vi "Read Temperature.vi"(0 "Session Handle in":T1, 11 "error in (no error)":errorcluster) -> (4 "Session Handle out":T1, 6 "Temperature":dbl, 8 "Success?":bool, 10 "Error Code":string, 15 "error out":errorcluster)   [LabVIEW 2015, in "PAS.lvclass"]
uses:
  PAS.lvclass
  Typedefs/Session Handle.ctl
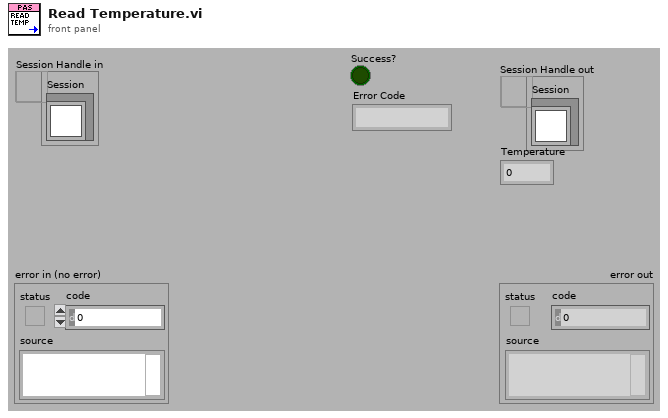
[diagram p1: front panel]
types:
  T1 = typedef "PAS.lvclass/Session Handle.ctl" = refnum<data-value>
  T2 = typedef "XNET Frame CAN.ctl" = cluster{"timestamp":timestamp, "payload":u8[], "identifier":u32, "type":T3, "extended?":bool, "echo?":bool}
  T3 = typedef "XNET Frame Type CAN.ctl" = u8
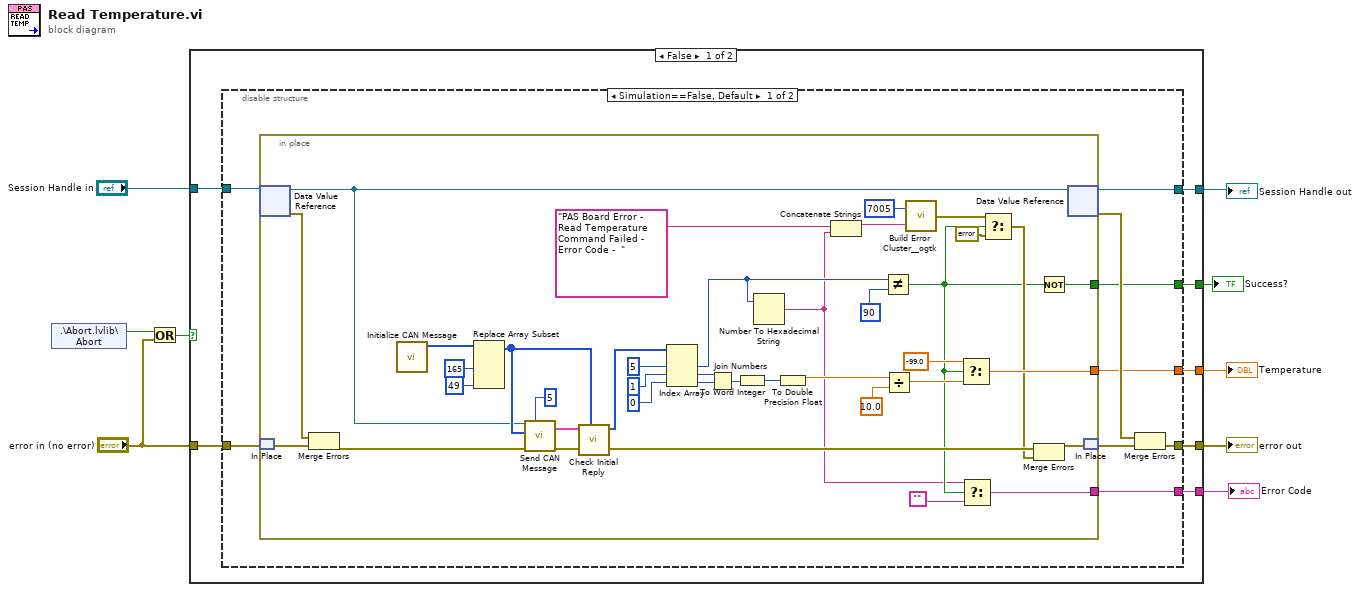
[diagram p0: block diagram]
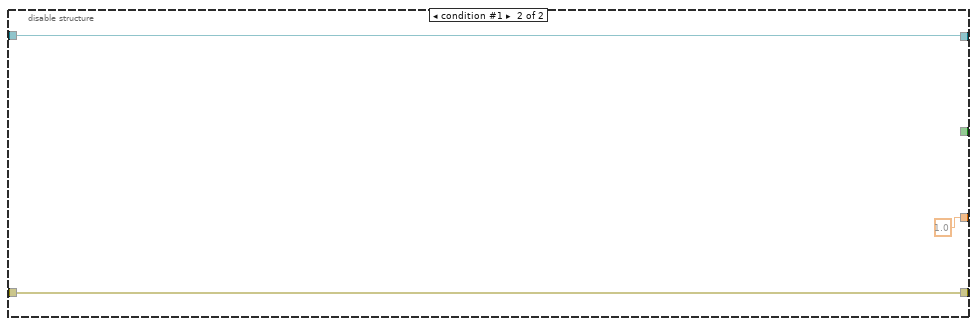
[diagram p2: hidden frame]
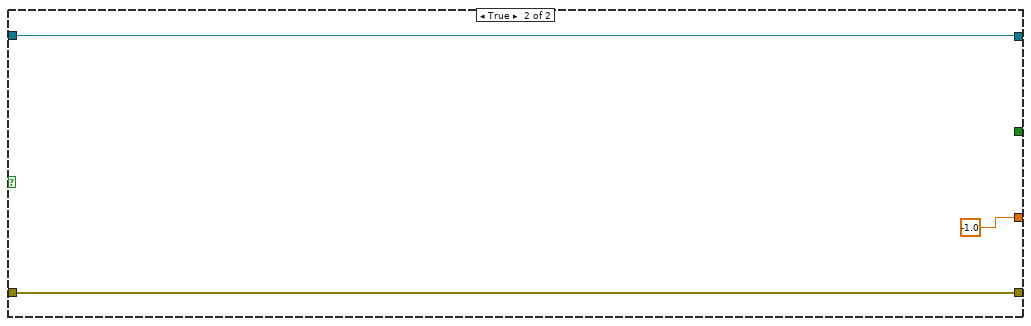
[diagram p3: hidden frame]
diagram:
  n1 = shared-variable ".\\Abort.lvlib\\Abort"() -> (w6:bool)  [unwired: 1 in, 1 out]
  n2 = Or(x=w6, y="error in (no error)") -> (x .or. y?=w4:bool)
  n3 = case shown="False" w4 {
    tunnel: [w16 w69] -> w8
    tunnel: [w15 w68] -> w7
    tunnel: "Session Handle in" -> [w14 w69]
    tunnel: "error in (no error)" -> [w13 w68]
    tunnel: [w12 -1.0] -> w3
    tunnel: [w11 _] -> w2
    tunnel: [w10 _] -> w1
    frame False {
      n4 = disable-structure shown="Simulation==False, Default" {
        disable-tunnel: [w25 w66] -> w16
        disable-tunnel: [w22 w65] -> w15
        disable-tunnel: w14 -> [w21 w66]
        disable-tunnel: w13 -> [w20 w65]
        disable-tunnel: [w19 1.0] -> w12
        disable-tunnel: [w18 _] -> w11
        disable-tunnel: [w17 _] -> w10
        frame condition #0 (active) {
          n5 = in-place {
            in-place-border: [w36] -> w19
            in-place-border: [w47] -> w18
            in-place-border: [w26] -> w17
            n6 = in-place-dvr #1(w21) -> (w54:refnum<class "PAS.lvclass">, w59:errorcluster)
            n7 = in-place-match #2(w20) -> (w58:errorcluster)
            n8 = Merge Errors(w59, w58) -> (w53:errorcluster)
            n9 = call "Initialize CAN Message.vi"() -> ("Initial Payload"=w61:u8[])  [unwired: 11 in]
            n10 = Replace Array Subset(array=w61, new element #1=u8 165 ("new element/subarray"), new element #2=u8 49 ("new element/subarray")) -> (w57:u8[])  [unwired: 2 in]
            n11 = call "Send CAN Message.vi"("Number of Retries"=5, "error in (no error)"=w53, "payload"=w57, "Gas In"=w54) -> ("error out"=w31:errorcluster, "Reply"=w55:T2[])  [unwired: 5 in, 1 out]
            n12 = call "Check Initial Reply.vi"("Write Message"=w57, "Reply"=w55) -> ("Data Packet"=w60:u8[])  [unwired: 7 in, 2 out]
            n13 = Index Array(array=w60, index #1=5 ("index"), index #2=1 ("index"), index #3=0 ("index")) -> (element #1=w48:u8, element #2=w43:u8, element #3=w42:u8)
            n14 = Join Numbers(hi=w43, lo=w42) -> ((hi.lo)=w41:u16)
            n15 = To Word Integer(number=w41) -> (16bit integer=w44:i16)
            n16 = Number To Hexadecimal String(2:w48) -> (0:w27:string)  [unwired: 1 in]
            n17 = To Double Precision Float(number=w44) -> (double precision float=w38:dbl)
            n18 = Concatenate Strings("PAS Board Error -  Read Temperature Command Failed - Error Code -  " ("string"), w27) -> (w51:string)
            n19 = Not Equal?(x=w48, y=u8 90 ("new element/subarray")) -> (x != y?=w28:bool)
            n20 = Divide(x=w38, y=10.0) -> (x/y=w33:dbl)
            n21 = call <userlib>:"Build Error Cluster__ogtk.vi"("String to Prepend to source (\"\")"=w51, "code"=7005) -> ("error out"=w40:errorcluster)
            n22 = Select(t=-99.0, s=w28, f=w33) -> (s? t:f=w36:dbl)
            n23 = Select(t=w27, s=w28, f="") -> (s? t:f=w26:string)
            n24 = Select(t=w40, s=w28, f=errorcluster {"status"=FALSE, "code"=0, "source"=""}) -> (s? t:f=w30:errorcluster)
            n25 = Merge Errors(w31, w30) -> (w62:errorcluster)
            n26 = Not(x=w28) -> (.not. x?=w47:bool)
            n27 = in-place-dvr #1(w54) -> (w25:T1, w23:errorcluster)
            n28 = in-place-match #2(w62) -> (w24:errorcluster)
          }
          n29 = Merge Errors(w23, w24) -> (w22:errorcluster)
        }
        frame condition #1 {
        }
      }
    }
    frame True {
    }
  }
  "Session Handle out" <- w8
  "error out" <- w7
  "Temperature" <- w3
  "Success?" <- w2
  "Error Code" <- w1
